vi "scan_dep_forloopfull duty back and forth_.vi"(0 "x range":dbl[](array[numeric]), 1 "Freq":dbl, 2 "error in":errorcluster, 3 "Mode":enum16{"Vertical", "Zigzag", "Horizontal"}(ring), 5 "y range":dbl[](array[numeric]), 7 "task/channels in":refnum<k21>, 9 "x pixels":dbl, 11 "y pixels":dbl, 12 "Time limit (s)":dbl) -> (6 "Progress":dbl(slide) scale=0.0..1.0, 8 "task out":refnum<k21>, 10 "Iterations":i32, 13 "error IO":errorcluster, 15 "Elapsed Time (s)":dbl)   [LabVIEW 2017]
uses:
  <vilib>/DAQmx/write.llb/DAQmx Write (Analog 1D Wfm NChan NSamp).vi
  <vilib>/DAQmx/configure/timing.llb/DAQmx Timing (Sample Clock).vi
  <vilib>/DAQmx/miscellaneous.llb/DAQmx Fill In Error Info.vi
panel:
  out "output array":dbl[](array[numeric])
  out "yvec":dbl[](array[numeric])
  out "xvec":dbl[](array[numeric])
  out "x*y":dbl
  out "nearest integer value":dbl
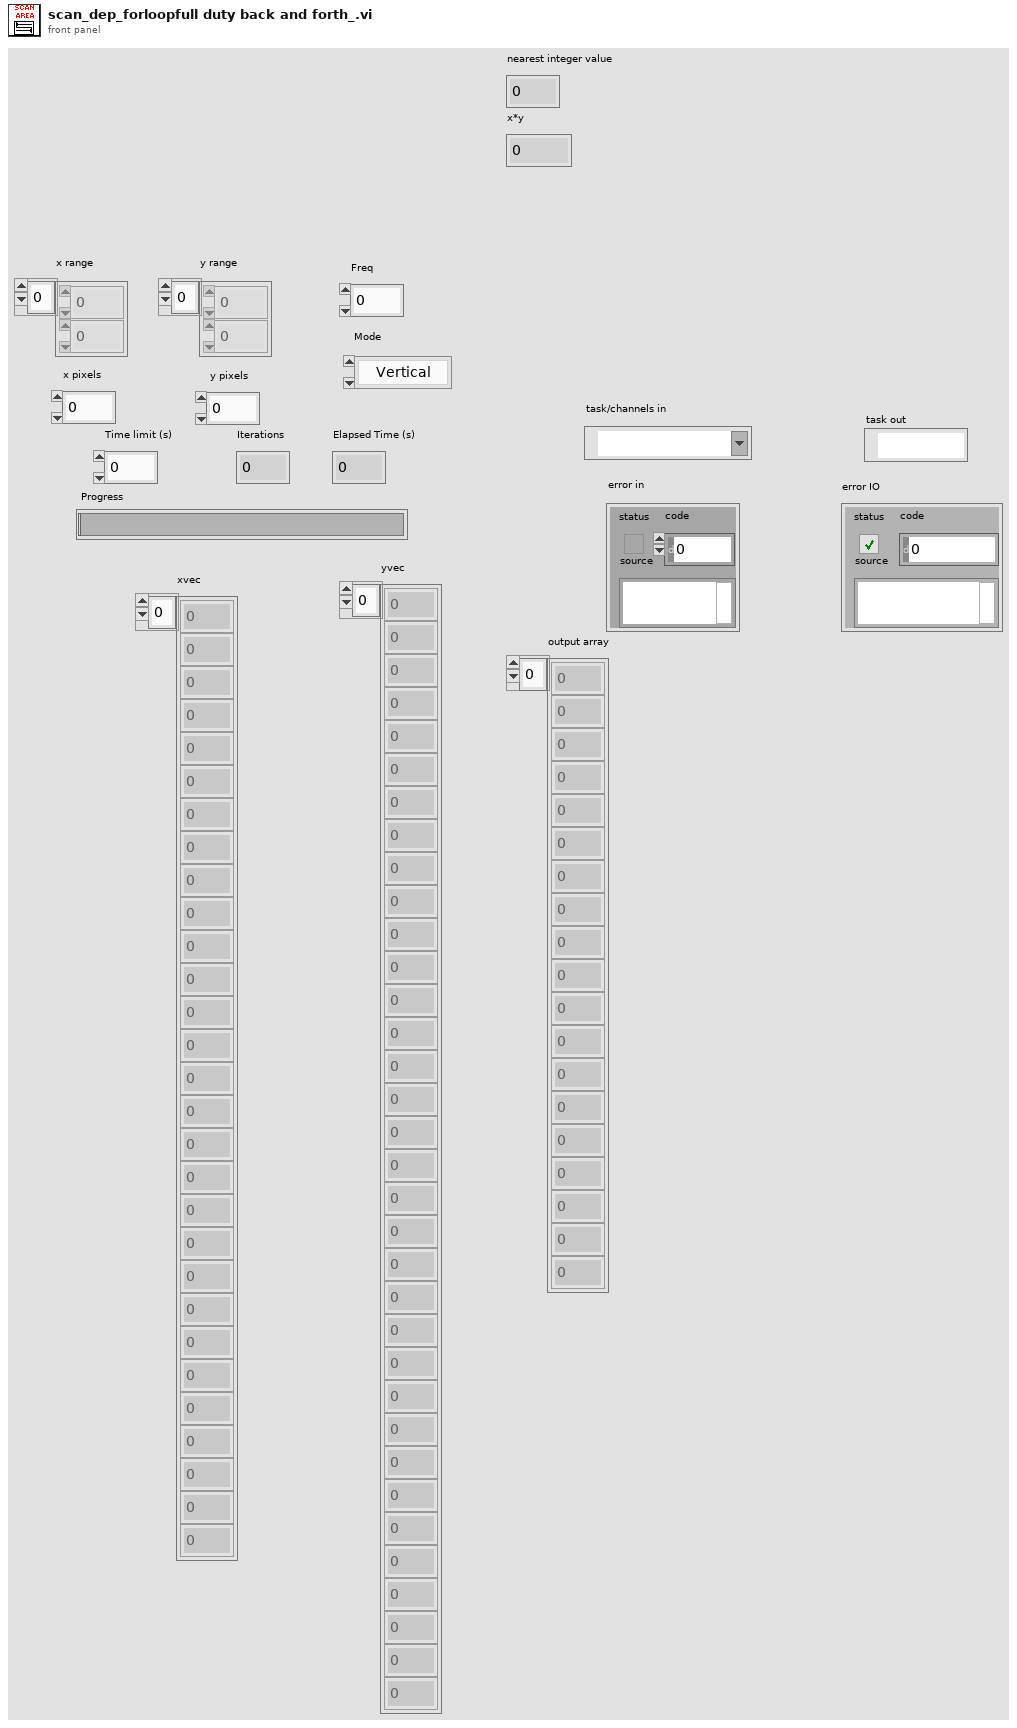
[diagram p1: front panel]
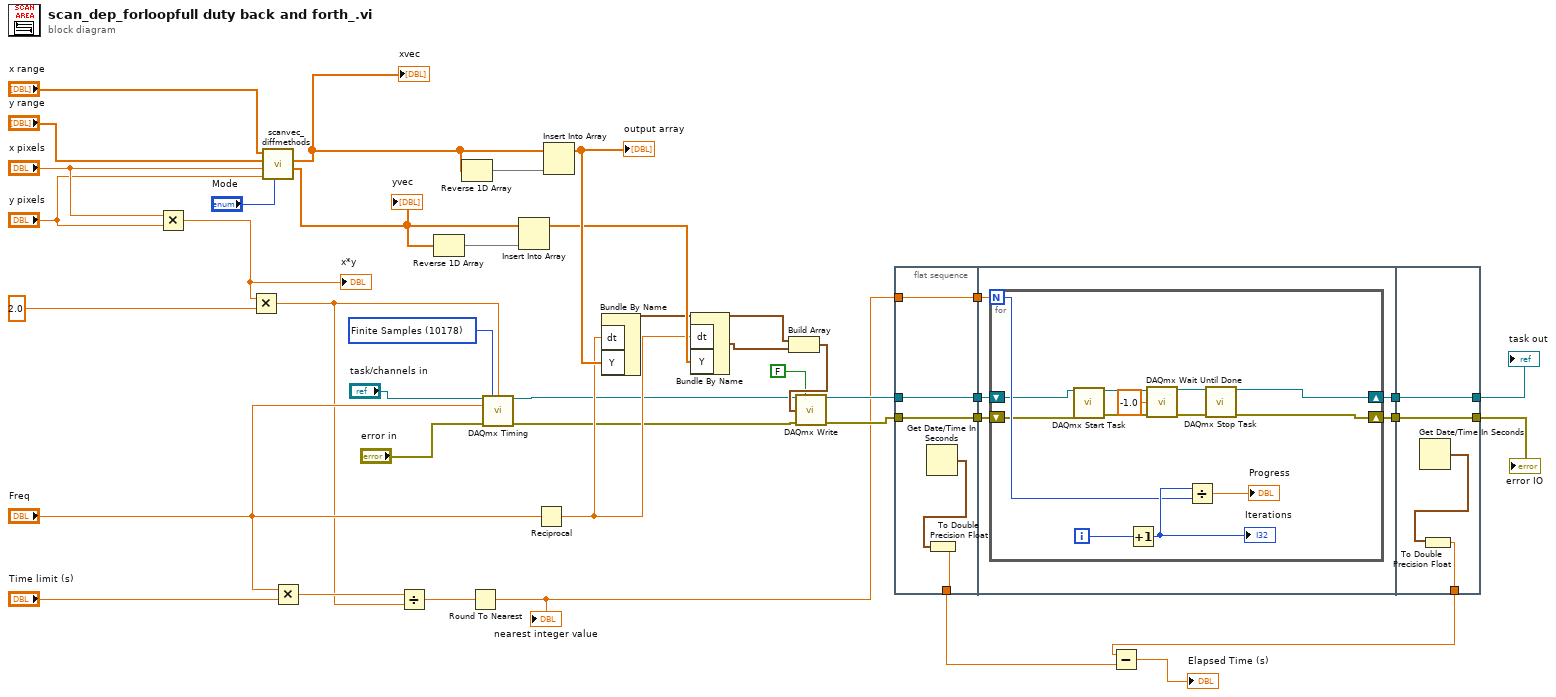
[diagram p0: block diagram]
diagram:
  w21 = 10178 items=["Finite Samples"=10178, "Continuous Samples"=10123, "Hardware Timed Single Point"=12522] ("sample mode")
  n1 = Multiply(x="x pixels", y="y pixels") -> (x*y=w34:dbl)
  "x*y" <- w34
  n2 = Multiply(x=w34, y=2.0) -> (x*y=w1:dbl)
  n3 = call "scanvec_diffmethods.vi"("Mode"="Mode", "y pixels"="y pixels", "x pixels"="x pixels", "y range"="y range", "x range"="x range") -> ("yvec"=w29:dbl[], "xvec"=w32:dbl[])  [unwired: 5 in]
  "xvec" <- w32
  "yvec" <- w29
  n4 = Multiply(x="Freq", y="Time limit (s)") -> (x*y=w12:dbl)
  n5 = Divide(x=w12, y=w1) -> (x/y=w14:dbl)
  n6 = Reverse 1D Array(array=w29) -> (reversed array=w27:dbl[])
  n7 = Reverse 1D Array(array=w32) -> (reversed array=w31:dbl[])
  n8 = Round To Nearest(number=w14) -> (nearest integer value=w11:dbl)
  "nearest integer value" <- w11
  n9 = call-poly <vilib>:"DAQmx Timing.vi"("task/channels in"="task/channels in", "sample mode"=w21, "samples per channel"=w1, "rate"="Freq", "error in"="error in") -> ("task out"=w2:refnum<k21>, "error out"=w3:errorcluster)  [unwired: 9 in]
  n10 = Insert Into Array(array=w29, new element=w27) -> (w28:dbl[])  [unwired: 1 in]
  n11 = Reciprocal(x="Freq") -> (1/x=w20:dbl)
  n12 = Insert Into Array(array=w32, new element=w31) -> (w30:dbl[])  [unwired: 1 in]
  "output array" <- w30
  n13 = Bundle By Name("dt"=w20, "Y"=w30) -> (w16:waveform(dbl))  [unwired: 1 in]
  n14 = Bundle By Name("dt"=w20, "Y"=w28) -> (w17:waveform(dbl))  [unwired: 1 in]
  n15 = Build Array(w16, w17) -> (w15:waveform(dbl)[])
  n16 = call-poly <vilib>:"DAQmx Write.vi"("task/channels in"=w2, "auto start"=FALSE, "data"=w15, "error in"=w3) -> ("task out"=w19:refnum<k21>, "error out"=w18:errorcluster)  [unwired: 9 in, 1 out]
  n17 = flat-sequence {
    tunnel: w11 -> [w45]
    tunnel: w18 -> [w42]
    tunnel: w19 -> [w46]
    tunnel: [w46] -> w26
    tunnel: [w42] -> w25
    tunnel: [w45] -> w24
    tunnel: [w43] -> w10
    tunnel: [w49] -> w23
    tunnel: [w48] -> w22
    tunnel: w26 -> [w51]
    tunnel: w25 -> [w50]
    tunnel: w24 -> [w47]
    tunnel: [w67] -> w41
    tunnel: [w68] -> w40
    tunnel: w23 -> [w68]
    tunnel: w22 -> [w67]
    tunnel: [w65] -> w9
    frame #0 {
      n18 = Get Date/Time In Seconds() -> (seconds since 1Jan1904=w44:timestamp)
      n19 = To Double Precision Float(number=w44) -> (double precision float=w43:dbl)
    }
    frame #1 {
      n20 = for {
        N: w47 -> [w60]
        shift-right: [w56] -> w48
        shift-left: w51 -> [w53]
        shift-right: [w54] -> w49
        shift-left: w50 -> [w58]
        i -> [w63]
        n21 = call <vilib>:"DAQmx Start Task.vi"("task/channels in"=w53, "error in"=w58) -> ("task out"=w64:refnum<k21>, "error out"=w59:errorcluster)  [unwired: 12 in]
        n22 = Increment(x=w63) -> (x+1=w61:i32)
        "Iterations" <- w61
        n23 = call <vilib>:"DAQmx Wait Until Done.vi"("task/channels in"=w64, "timeout (sec)"=-1.0, "error in"=w59) -> ("task out"=w57:refnum<k21>, "error out"=w55:errorcluster)  [unwired: 11 in]
        n24 = Divide(x=w61, y=w60) -> (x/y=→"Progress":dbl)
        n25 = call <vilib>:"DAQmx Stop Task.vi"("task/channels in"=w57, "error in"=w55) -> ("task out"=w56:refnum<k21>, "error out"=w54:errorcluster)  [unwired: 12 in]
      }
    }
    frame #2 {
      n26 = Get Date/Time In Seconds() -> (seconds since 1Jan1904=w66:timestamp)
      n27 = To Double Precision Float(number=w66) -> (double precision float=w65:dbl)
    }
  }
  n28 = Subtract(x=w9, y=w10) -> (x-y=→"Elapsed Time (s)":dbl)
  "task out" <- w41
  "error IO" <- w40
